vi "Handle Command.vi"(8 "error in":errorcluster, 10 "Change iSpkEn in":refnum<class "Change iSpk Signal.lvclass">, 11 "Object In":refnum<class>) -> (0 "error out":errorcluster, 1 "Command Successful?":bool, 2 "Change iSpkEn out":refnum<class "Change iSpk Signal.lvclass">, 3 "Object Out":refnum<class>)   [LabVIEW 2014, in "ePAS Library.lvlib" / "Change iSpk Signal.lvclass"]
doc: "Abstract method for accomplishing the execution of a command directed to an instrument object on the wire."
uses:
  Change iSpk Signal.lvclass
  Instrument/ePAS.lvclass
  Instrument/ePAS.lvclass/ePAS.ctl
  Change iSpk Signal.lvclass/Change iSpk Signal.ctl
  <vilib>/Utility/error.llb/Error Cluster From Error Code.vi
  <vilib>/rvi/errors/niLvFpgaAdjustHostInterfaceError.vi
  <vilib>/rvi/interface/nirviReadWriteControl/nirviReadWriteControl.xnode
  FPGA/R FPGA Ref.ctl
  FPGA Bitfiles/FPGA Server.lvbitx
  FPGA/Session/Exscalabar FPGA.lvclass
  ePAS Library.lvlib
  NiFpgaLv.dll
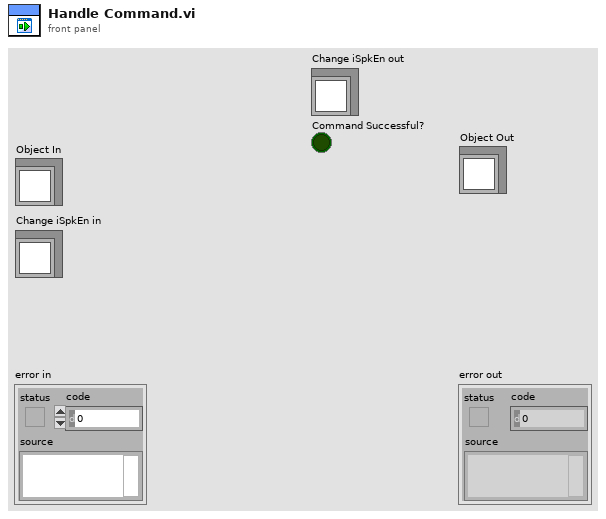
[diagram p1: front panel]
types:
  T1 = typedef "Session - Root.lvclass/Session Handle.ctl" = refnum<data-value>
  T2 = typedef "ePAS Library.lvlib/R FPGA Ref.ctl" = refnum<k20>
  T3 = cluster{"iSpkEn[0]":bool, "iSpkEn[1]":bool, "iSpkEn[2]":bool, "iSpkEn[3]":bool, "iSpkEn[4]":bool}
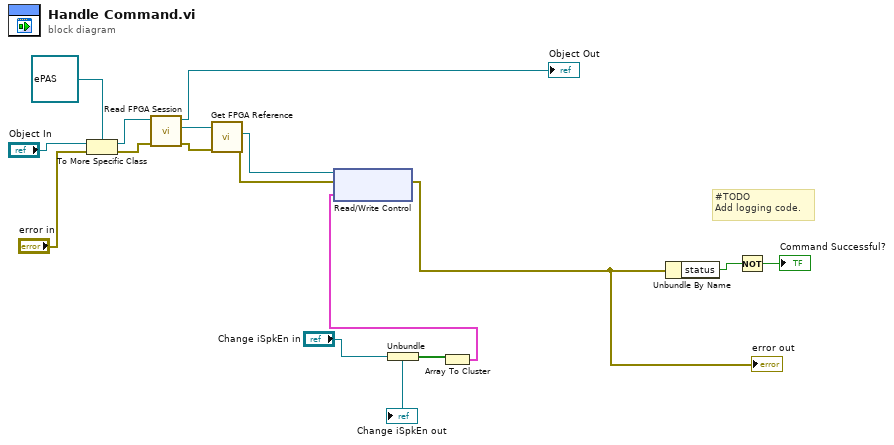
[diagram p0: block diagram]
diagram:
  # "#TODO\nAdd logging code."
  n1 = To More Specific Class(target class=refnum<class "ePAS.lvclass"> refnum ("ePAS"), reference="Object In", error in="error in") -> (specific class reference=w14:refnum<class "ePAS.lvclass">, error out=w13:errorcluster)
  n2 = call "Read FPGA Session.vi"("error in (no error)"=w13, "ePAS in"=w14) -> ("error out"=w9:errorcluster, "Session Handle"=w12:T1, "ePAS out"=→"Object Out":refnum<class "ePAS.lvclass">)  [unwired: 7 in]
  n3 = call "Get FPGA Reference.vi"("error in"=w9, "Session In"=w12) -> ("error out"=w7:errorcluster, "Ex FPGA Ref"=w11:T2)  [unwired: 7 in, 1 out]
  n4 = Unbundle("Change iSpkEn in") -> (w4:bool[])
  n5 = Array To Cluster(array=w4) -> (cluster=w6:T3)
  n6 = xnode "Read/Write Control"("FPGA VI Reference In"=w11, "error in"=w7, "iSpk Enable"=w6) -> ("error out"=w3:errorcluster)  [unwired: 1 out]
  "error out" <- w3
  n7 = Unbundle By Name(w3) -> ("status"=w2:bool)
  n8 = Not(x=w2) -> (.not. x?=→"Command Successful?":bool)
  "Change iSpkEn out" <- "Change iSpkEn in"
